vi "json_is_null.vi"(1 "variant in":variant) -> (0 "is_null?":bool)   [LabVIEW 2017, in "rethinkdb.lvlib"]
uses:
  rethinkdb.lvlib
  <vilib>/Utility/Data Type/NI_Data Type.lvlib
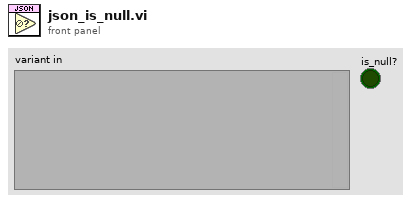
[diagram p1: front panel]
types:
  T1 = typedef "NI_Data Type.lvlib/Data Type.ctl" = enum8{"Invalid Type", "Void", "I8", "I16", "I32", "I64", "U8", "U16", "U32", "U64", "Single Float", "Double Float", "Extended Float", "Single Complex", "Double Complex", "Extended Complex", "Enum U8", "Enum U16", "Enum U32", "Enum U64", "Single Float With Unit", "Double Float With Unit", "Extended Float With Unit", "Single Complex with Unit", "Double Complex with Unit", "Extended Complex with Unit", "Boolean", "String", "Path", "Picture", "Tag", "Array", "Cluster", "Variant", "LV Variant", "Waveform", "Timestamp", "Digital Waveform", "Digital Data", "ExpressData", "Refnum", "External Data", "VI", "Poly VI", "LabVIEW Class Instance", "Fixed Point"}
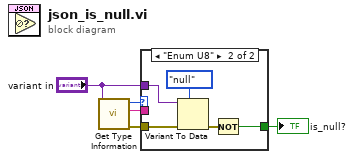
[diagram p0: block diagram]
diagram:
  n1 = call <vilib>:"Get Type Information.vi"("Variant"="variant in") -> ("error out"=w4:errorcluster, "Name"=w2:string, "Type"=w3:T1)  [unwired: 6 in, 2 out]
  n2 = case shown="\"Enum U8\"" w3 {
    tunnel: w4 -> [_ w10]
    tunnel: "variant in" -> [_ w9]
    tunnel: w2 -> [_ _]
    tunnel: [_ w6] -> w1
    frame Default {
    }
    frame "Enum U8" {
      n3 = Variant To Data(error in=w10, type=enum8{"null"}."null", Variant=w9) -> (error out=w7:errorcluster)  [unwired: 1 out]
      n4 = Not(x=w7) -> (.not. x?=w6:bool)
    }
  }
  "is_null?" <- w1
